vi "Secure-Release Region.vi"(7 "Action":enum16{"Secure", "Release"}(ring), 8 "error in (no error)":errorcluster, 10 "Control In":T1={"I-O.lvclass"=refnum, "Gantry"=refnum, "Dispenser"="COM1"}, 11 "Workspace in":refnum<class "Component Tray.lvclass">) -> (0 "error out":errorcluster, 2 "Control Out":T1={"I-O.lvclass"=refnum, "Gantry"=refnum, "Dispenser"="COM1"}, 3 "Workspace out":refnum<class "Component Tray.lvclass">)   [LabVIEW 2020, in "Component Tray.lvclass"]
uses:
  Component Tray.lvclass
  Controller/I-O/I-O.lvclass
  Fixture.lvclass
  Controller/Controllers.ctl
  Controller/Controller.lvclass
  C:/Program Files (x86)/Aerotech/A3200/LabVIEW/2010/Bin/Aerotech.A3200.dll
  Program Files (x86)/Aerotech/A3200/LabVIEW/2010/Bin/Aerotech.A3200.dll
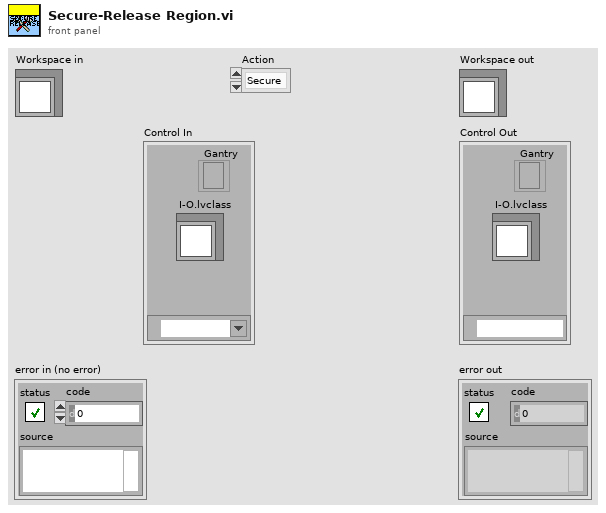
[diagram p1: front panel]
types:
  T1 = typedef "Controller.lvclass/Controllers.ctl" = cluster{"I-O.lvclass":refnum<class "I-O.lvclass">, "Gantry":refnum<k24>, "Dispenser":refnum<visa-resource-name>}
  T2 = typedef "I-O.lvclass/Pin Map.ctl" = cluster{"Region Valves":i32[], "Extra Valves":dbl[][][], "Tool Primary Valve":i32, "Tool Secondary Valve":i32, "Region Sensors":i32[], "Extra Sensors":dbl[][][], "Tool Primary Sensor":dbl, "Tool Secondary Sensor":dbl, "Compression Sensor":dbl, "5V":i32, "Dispenser Sensor":dbl}
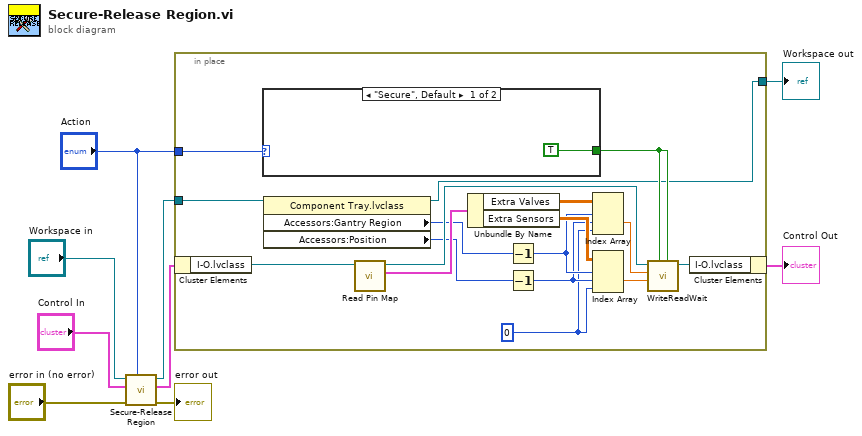
[diagram p0: block diagram]
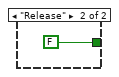
[diagram p2: hidden frame]
diagram:
  n1 = call-parent "Secure-Release Region.vi"("Action"="Action", "error in (no error)"="error in (no error)", "Control In"="Control In", "Fixture in"="Workspace in") -> ("error out"=→"error out":errorcluster, "Control Out"=w5:T1, "Fixture out"=w2:refnum<class "Component Tray.lvclass">)  [unwired: 5 in]
  n2 = in-place {
    in-place-border: "Action" -> [w23]
    in-place-border: w2 -> [w20]
    in-place-border: [w13] -> w1
    w10 = 0
    n3 = in-place-cluster #1(w5) -> ("I-O.lvclass"=w25:refnum<class "I-O.lvclass">)
    n4 = case shown="\"Secure\", Default" w23 {
      tunnel: [TRUE FALSE] -> w24
      frame "Secure", Default {
      }
      frame "Release" {
      }
    }
    n5 = property class="Component Tray.lvclass"(reference=w20) -> (reference out=w13:refnum<class "Component Tray.lvclass">, "Accessors:Gantry Region"=w17:i32, "Accessors:Position"=w15:i32)  [unwired: 1 in, 1 out]
    n6 = call-dynamic "Read Pin Map.vi"("I-O in"=w25) -> ("Pin Map 2"=w26:T2, "I-O out"=w22:refnum<class "I-O.lvclass">)  [unwired: 8 in, 1 out]
    n7 = Unbundle By Name(w26) -> ("Extra Valves"=w19:dbl[][][], "Extra Sensors"=w18:dbl[][][])
    n8 = Decrement(x=w17) -> (x-1=w16:i32)
    n9 = Decrement(x=w15) -> (x-1=w14:i32)
    n10 = Index Array(array=w19, index (dim 0)=w16, index (dim 1)=w14, index (dim 2)=w10) -> (element=w12:dbl)
    n11 = Index Array(array=w18, index (dim 0)=w16, index (dim 1)=w14, index (dim 2)=w10) -> (element=w11:dbl)
    n12 = call "WriteReadWait.vi"("Read Value"=w24, "Write Value"=w24, "Read"=w11, "Write"=w12, "I-O in"=w22) -> ("I-O out"=w21:refnum<class "I-O.lvclass">)  [unwired: 5 in, 1 out]
    n13 = in-place-cluster #1("I-O.lvclass"=w21) -> (→"Control Out":T1)
  }
  "Workspace out" <- w1
